vi "Update UI per Reference.vi"(8 "error in (no error)":errorcluster, 11 "Analyze Compound Results Base in":refnum<class "Analyze Compound Results Base.lvclass">) -> (0 "error out":errorcluster, 3 "Analyze Compound Results Base out":refnum<class "Analyze Compound Results Base.lvclass">)   [LabVIEW 2020, in "Analyze Compound Results Base.lvclass"]
uses:
  Analyze Compound Results Base.lvclass
  Analyze Compound Results Base.lvclass/Analyze Compound Results Base.ctl
  Results Base/Analyze Results Base.lvclass
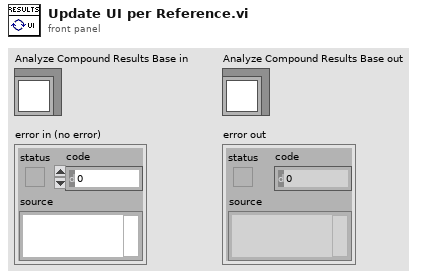
[diagram p1: front panel]
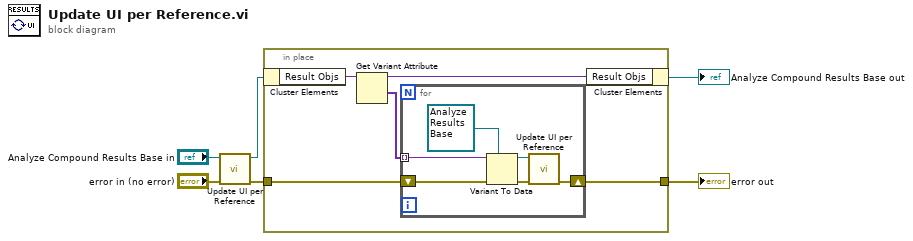
[diagram p0: block diagram]
diagram:
  n1 = call-parent "Update UI per Reference.vi"("error in (no error)"="error in (no error)", "Analyze Results Base in"="Analyze Compound Results Base in") -> ("error out"=w4:errorcluster, "Analyze Results Base out"=w3:refnum<class "Analyze Compound Results Base.lvclass">)  [unwired: 8 in]
  n2 = in-place {
    in-place-border: w4 -> [w8]
    in-place-border: [w7] -> w1
    n3 = in-place-cluster #1(w3) -> ("Result Objs"=w11:variant)
    n4 = Get Variant Attribute(Variant=w11) -> (duplicate Variant=w10:variant, values=w9:variant[])  [unwired: 3 in, 2 out]
    n5 = for {
      tunnel: w9 -> [w17] mode=indexing
      shift-right: [w13] -> w7
      shift-left: w8 -> [w14]
      n6 = Variant To Data(error in=w14, type=refnum<class "Analyze Results Base.lvclass"> refnum ("Analyze Results Base.lvclass"), Variant=w17) -> (data=w15:refnum<class "Analyze Results Base.lvclass">, error out=w12:errorcluster)
      n7 = call-dynamic "Update UI per Reference.vi"("error in (no error)"=w12, "Analyze Results Base in"=w15) -> ("error out"=w13:errorcluster)  [unwired: 8 in, 1 out]
    }
    n8 = in-place-cluster #1("Result Objs"=w10) -> (→"Analyze Compound Results Base out":refnum<class "Analyze Compound Results Base.lvclass">)
  }
  "error out" <- w1
